vi "Tree.vi"   [LabVIEW 2017]
doc: "Tree diagram for CLAUDIE_xlsx"
uses:
  <vilib>/ATEsystem/CLAUDIE_xlsx/Excel_class/Excel_class.lvclass
  <vilib>/ATEsystem/CLAUDIE_xlsx/Excel_class/Insert_data/Insert Element.vi
  <vilib>/ATEsystem/CLAUDIE_xlsx/Excel_class/New xlsx.vi
  <vilib>/ATEsystem/CLAUDIE_xlsx/Excel_class/Formating/Set Style All.vi
panel:
  # "ATEsystem"
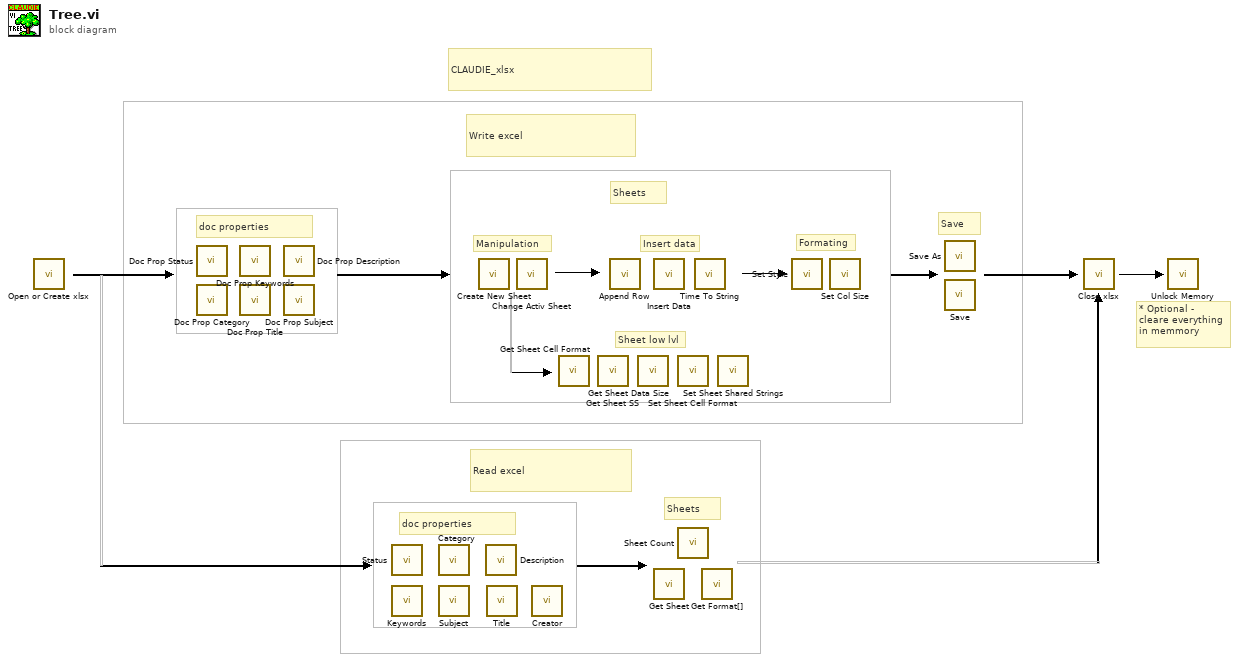
[diagram p0: block diagram]
diagram:
  # "CLAUDIE_xlsx"
  # "Save"
  # "Sheets"
  # "Read excel"
  # "doc properties"
  # "* Optional - \ncleare everything\nin memmory"
  # "Write excel"
  # "Sheets"
  # "doc properties"
  # "Sheet low lvl"
  # "Manipulation"
  # "Formating"
  # "Insert data"
  n1 = call-poly <vilib>:"Open or Create xlsx.vi"() -> ()  [unwired: 10 in, 2 out]
  n2 = call <vilib>:"Doc Prop Status.vi"() -> ()  [unwired: 10 in, 2 out]
  n3 = call <vilib>:"Doc Prop Category.vi"() -> ()  [unwired: 10 in, 2 out]
  n4 = call <vilib>:"Doc Prop Keywords.vi"() -> ()  [unwired: 10 in, 2 out]
  n5 = call <vilib>:"Doc Prop Title.vi"() -> ()  [unwired: 10 in, 2 out]
  n6 = call <vilib>:"Doc Prop Description.vi"() -> ()  [unwired: 10 in, 2 out]
  n7 = call <vilib>:"Doc Prop Subject.vi"() -> ()  [unwired: 10 in, 2 out]
  n8 = call <vilib>:"Status.vi"() -> ()  [unwired: 9 in, 3 out]
  n9 = call <vilib>:"Keywords.vi"() -> ()  [unwired: 9 in, 3 out]
  n10 = call <vilib>:"Category.vi"() -> ()  [unwired: 9 in, 3 out]
  n11 = call <vilib>:"Subject.vi"() -> ()  [unwired: 9 in, 3 out]
  n12 = call <vilib>:"Create New Sheet.vi"() -> ()  [unwired: 9 in, 3 out]
  n13 = call <vilib>:"Description.vi"() -> ()  [unwired: 9 in, 3 out]
  n14 = call <vilib>:"Title.vi"() -> ()  [unwired: 9 in, 3 out]
  n15 = call <vilib>:"Change Activ Sheet.vi"() -> ()  [unwired: 9 in, 3 out]
  n16 = call <vilib>:"Creator.vi"() -> ()  [unwired: 9 in, 3 out]
  n17 = call <vilib>:"Get Sheet Cell Format.vi"() -> ()  [unwired: 8 in, 4 out]
  n18 = call <vilib>:"Get Sheet SS.vi"() -> ()  [unwired: 8 in, 4 out]
  n19 = call <vilib>:"Append Row.vi"() -> ()  [unwired: 8 in, 4 out]
  n20 = call <vilib>:"Get Sheet Data Size.vi"() -> ()  [unwired: 8 in, 4 out]
  n21 = call-poly <vilib>:"Insert Data.vi"() -> ()  [unwired: 9 in, 3 out]
  n22 = call <vilib>:"Get Sheet.vi"() -> ()  [unwired: 8 in, 4 out]
  n23 = call <vilib>:"Set Sheet Cell Format.vi"() -> ()  [unwired: 9 in, 3 out]
  n24 = call <vilib>:"Sheet Count.vi"() -> ()  [unwired: 8 in, 4 out]
  n25 = call <vilib>:"Time To String.vi"() -> ()  [unwired: 1 in, 1 out]
  n26 = call <vilib>:"Get Format[].vi"() -> ()  [unwired: 9 in, 3 out]
  n27 = call <vilib>:"Set Sheet Shared Strings.vi"() -> ()  [unwired: 9 in, 3 out]
  n28 = call-poly <vilib>:"Set Style.vi"() -> ()  [unwired: 9 in, 3 out]
  n29 = call <vilib>:"Set Col Size.vi"() -> ()  [unwired: 10 in, 2 out]
  n30 = call <vilib>:"Save As.vi"() -> ()  [unwired: 10 in, 2 out]
  n31 = call <vilib>:"Save.vi"() -> ()  [unwired: 10 in, 2 out]
  n32 = call <vilib>:"Close xlsx.vi"() -> ()  [unwired: 11 in, 1 out]
  n33 = call <vilib>:"Unlock Memory.vi"() -> ()  [unwired: 11 in, 1 out]
